vi "Step Get All By Test Type.vi"(8 "error in (no error)":errorcluster, 10 "sxTestId (\"\")":string, 11 "Connection Refnum":T1) -> (0 "error out":errorcluster, 2 "Sequence Steps":T2[](array[typedef]), 3 "Connection Refnum":T1, 4 "Data Present":bool)   [LabVIEW 2011]
uses:
  Step Record.ctl
  SI.LIB/ODBC/SQL Controls/Connection Refnum.ctl
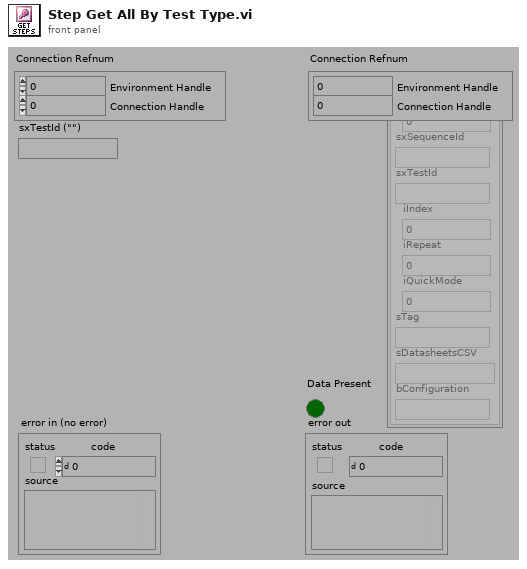
[diagram p1: front panel]
types:
  T1 = typedef "Connection Refnum.ctl" = cluster{"Environment Handle":i32, "Connection Handle":i32}
  T2 = typedef "Step Record.ctl" = cluster{"ixStep":i32, "sxSequenceId":string, "sxTestId":string, "iIndex":i32, "iRepeat":i32, "iQuickMode":i32, "sTag":string, "sDatasheetsCSV":string, "bConfiguration":string}
  T3 = typedef "Statement Refnum.ctl" = cluster{"Statement Handle":i32, "Parameter Number":u16}
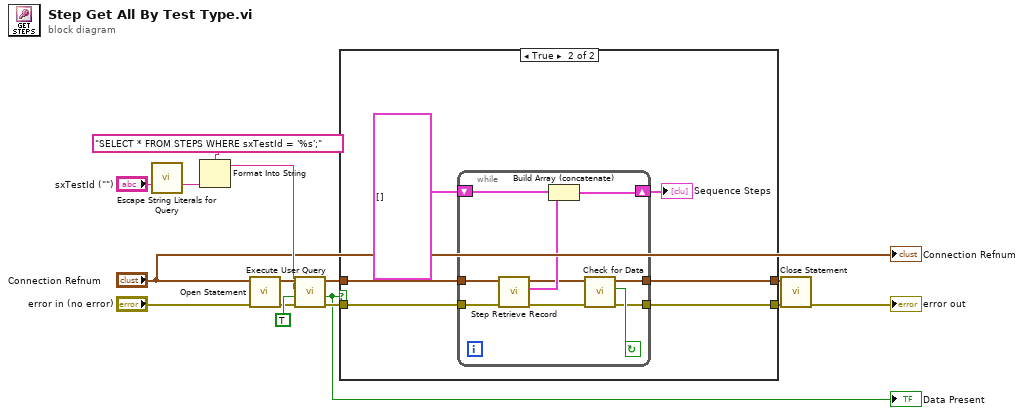
[diagram p0: block diagram]
diagram:
  n1 = call "Escape String Literals for Query.vi"("String"="sxTestId (\"\")") -> ("escaped String"=w1:string)  [unwired: 1 in, 13 out]
  n2 = Format Into String(format string="SELECT * FROM STEPS WHERE sxTestId = '%s';" ("User Query"), w1) -> (resulting string=w8:string)  [unwired: 2 in, 1 out]
  n3 = call "Open Statement.vi"("error in (no error)"="error in (no error)", "Connection Refnum"="Connection Refnum") -> ("error out"=w9:errorcluster, "Statement Refnum"=w10:T3)  [unwired: 4 out]
  n4 = call "Execute User Query.vi"("error in (no error)"=w9, "Return Data? (f)"=TRUE, "User Query"=w8, "Statement Refnum"=w10) -> ("error out"=w15:errorcluster, "Data Present?"=w7:bool, "Statement Refnum"=w14:T3)  [unwired: 1 out]
  "Data Present" <- w7
  n5 = case shown="True" w7 {
    tunnel: w15 -> [w16 w22]
    tunnel: w14 -> [w17 w23]
    tunnel: [w16 w20] -> w11
    tunnel: [w17 w21] -> w12
    frame False {
    }
    frame True {
      n6 = while {
        tunnel: w23 -> [w29]
        tunnel: w22 -> [w28]
        tunnel: [w26] -> w21
        tunnel: [w24] -> w20
        shift-right: [w33] -> w18
        shift-left: T2[] [] -> [w32]
        stop <- w31 continue-if-true
        n7 = call "Step Retrieve Record.vi"("error in (no error)"=w28, "Statement Refnum"=w29) -> ("error out"=w25:errorcluster, "Step"=w30:T2, "Statement Refnum"=w27:T3)  [unwired: 7 out]
        n8 = Build Array (concatenate)(w32, w30) -> (w33:T2[])
        n9 = call "Check for Data.vi"("error in (no error)"=w25, "Statement Refnum"=w27) -> ("error out"=w24:errorcluster, "Data Present?"=w31:bool, "Statement Refnum"=w26:T3)  [unwired: 3 out]
      }
      "Sequence Steps" <- w18
    }
  }
  n10 = call "Close Statement.vi"("error in (no error)"=w11, "Statement Refnum"=w12) -> ("error out"=→"error out":errorcluster)  [unwired: 5 out]
  "Connection Refnum" <- "Connection Refnum"
